vi "lidar_plot.vi"(0 "LiDAR Data":T2(array[cluster]), 1 "Number points":i32=14400, 2 "error in":errorcluster) -> (3 "LiDAR points":sgl[][](array[numeric]), 4 "Intensity":u8[](array[numeric]), 6 "error out":errorcluster)   [LabVIEW 2019, in "Lib_Simx.lvlib"]
doc: "Plot Lidar data into a 3D Plot Datatype.lvclass."
uses:
  Lib_Simx.lvlib
  <vilib>/Utility/miscctls.llb/LVRGBAColorTypeDef.ctl
panel:
  in  "Plot Lidar":bool=TRUE
  out "Laser Returns":i32
  out "Color Map":dbl[][](graph)
  out "Intensity(0-255)":T1[](array[typedef])
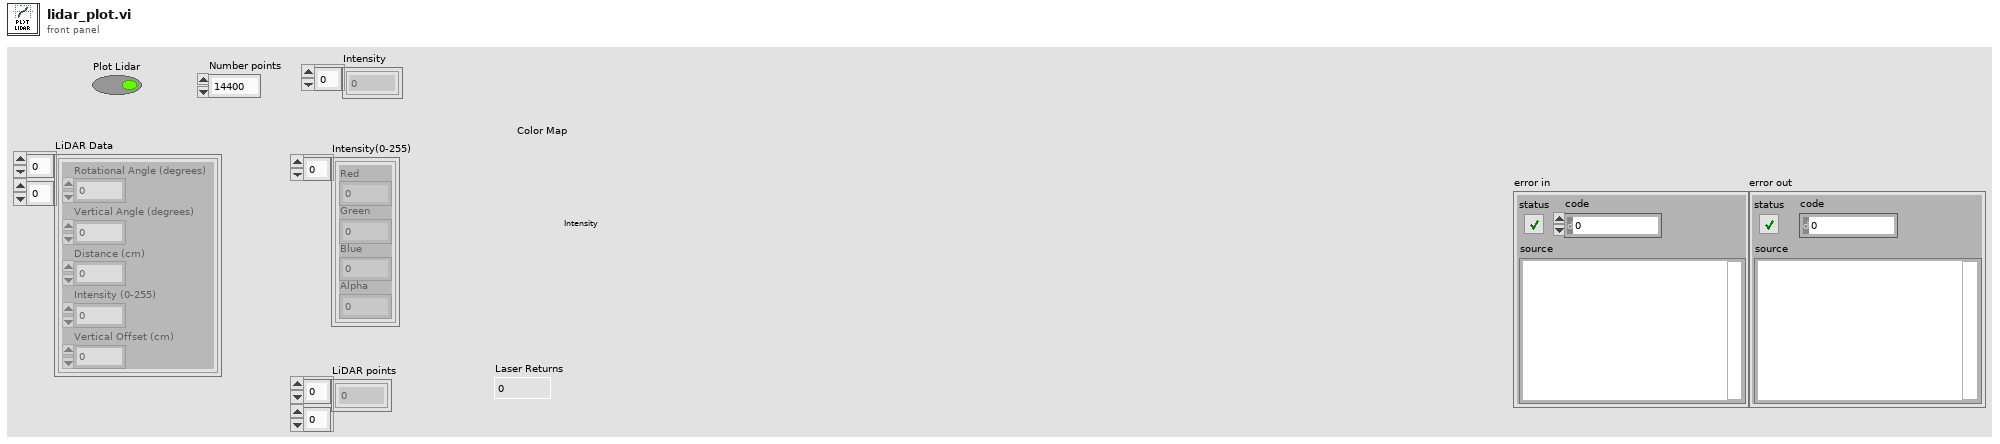
[diagram p1: front panel]
types:
  T1 = typedef "LVRGBAColorTypeDef.ctl" = cluster{"Red":sgl, "Green":sgl, "Blue":sgl, "Alpha":sgl}
  T2 = cluster{"Rotational Angle (degrees)":dbl, "Vertical Angle (degrees)":dbl, "Distance (cm)":dbl, "Intensity (0-255)":u8, "Vertical Offset (cm)":dbl}[][]
  T3 = cluster{"Rotational Angle (degrees)":dbl, "Vertical Angle (degrees)":dbl, "Distance (cm)":dbl, "Intensity (0-255)":u8, "Vertical Offset (cm)":dbl}[]
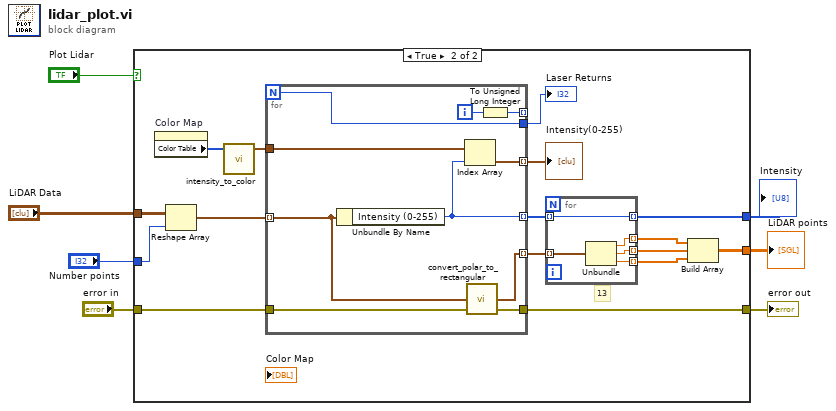
[diagram p0: block diagram]
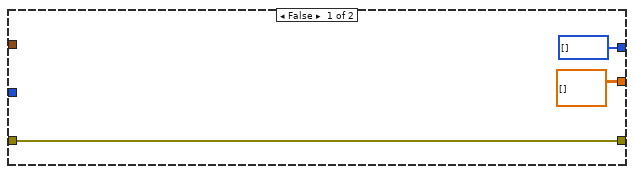
[diagram p2: hidden frame]
diagram:
  n1 = case shown="True" "Plot Lidar" {
    tunnel: "LiDAR Data" -> [_ w26]
    tunnel: "error in" -> [w10 w19]
    tunnel: [w10 w18] -> w4
    tunnel: [sgl[][] [] w14] -> w3
    tunnel: "Number points" -> [_ w13]
    tunnel: [u8[] [] w11] -> w1
    frame False {
    }
    frame True {
      # "13"
      n2 = property on="Color Map" class="IntGraph (strict)"() -> ("Color Table"=w21:u32[])  [unwired: 2 in, 2 out]
      n3 = Reshape Array(w26, w13) -> (w25:T3)
      n4 = call "intensity_to_color.vi"("Color Table"=w21) -> ("RGBA array"=w20:T1[])  [unwired: 4 in]
      n5 = for {
        N -> [w39]
        tunnel: [w35] -> w23 mode=indexing
        tunnel: [w38] -> w22 mode=indexing
        tunnel: [w40] -> _ mode=indexing
        tunnel: [w39] -> w24
        tunnel: w20 -> [w37]
        tunnel: w25 -> [w36] mode=indexing
        tunnel: w19 -> [w34]
        tunnel: [w33] -> w18
        tunnel: [w32] -> w12 mode=indexing
        i -> [w41]
        n6 = Unbundle By Name(w36) -> ("Intensity (0-255)"=w32:u8)
        n7 = Index Array(array=w37, index=w32) -> (element=w38:T1)
        n8 = call "convert_polar_to_rectangular.vi"("error in"=w34, "Laser Packet"=w36) -> ("error out"=w33:errorcluster, "Cartesian Coordinates"=w35:cluster{"X":sgl, "Y":sgl, "Z":sgl})  [unwired: 2 in]
        n9 = To Unsigned Long Integer(number=w41) -> (unsigned 32bit integer=w40:u32)
      }
      "Laser Returns" <- w24
      "Intensity(0-255)" <- w22
      n10 = for {
        tunnel: w23 -> [w31] mode=indexing
        tunnel: [w30] -> w17 mode=indexing
        tunnel: [w29] -> w16 mode=indexing
        tunnel: [w28] -> w15 mode=indexing
        tunnel: w12 -> [w27] mode=indexing
        tunnel: [w27] -> w11 mode=indexing
        n11 = Unbundle(w31) -> ("X"=w30:sgl, "Y"=w29:sgl, "Z"=w28:sgl)
      }
      n12 = Build Array(w17, w16, w15) -> (w14:sgl[][])
    }
  }
  "error out" <- w4
  "LiDAR points" <- w3
  "Intensity" <- w1
